vi "lib Compare Files in Folder.vi"() -> ()   [LabVIEW 2011]
panel:
  out "Array":T1(array[cluster])
  out "Horizontal Graduated Bar":u8(slide) scale=0.0..100.0
  out "All Files in Dir":path[](array[path])
  in  "Folder Path 2":path
  in  "Folder Path":path
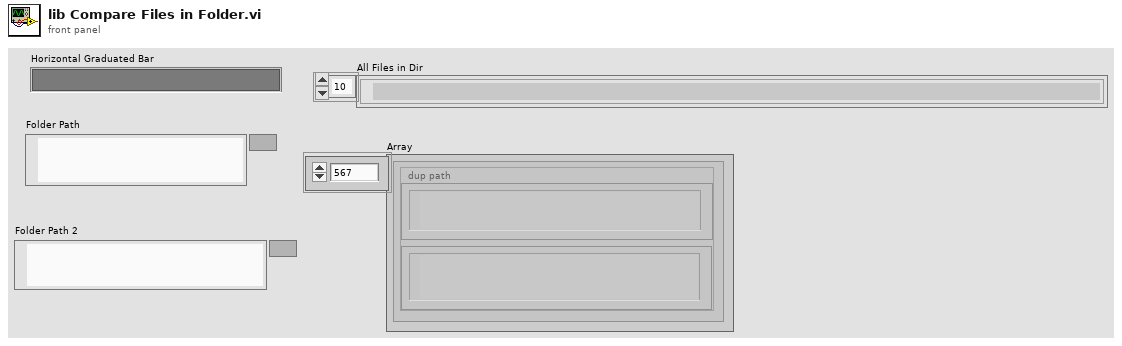
[diagram p1: front panel]
types:
  T1 = cluster{"dup path":path, "File Path Control":path}[]
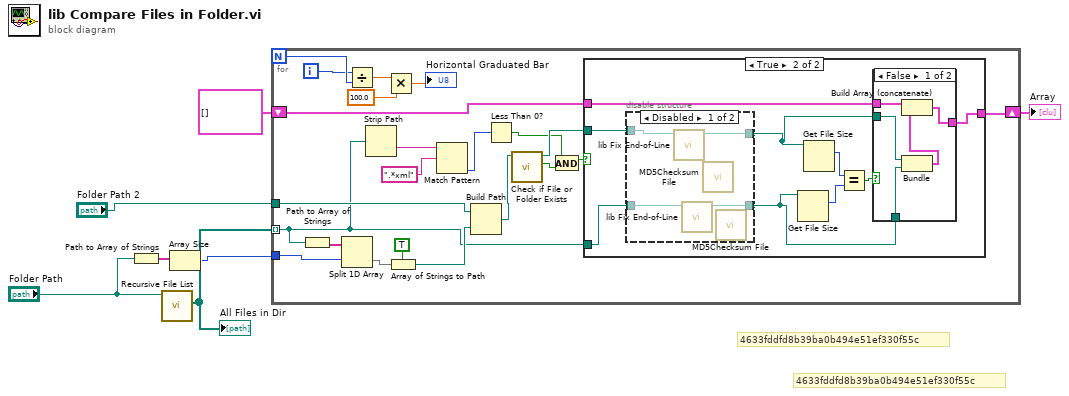
[diagram p0: block diagram]
diagram:
  # "4633fddfd8b39ba0b494e51ef330f55c"
  # "4633fddfd8b39ba0b494e51ef330f55c"
  n1 = Path to Array of Strings(0:"Folder Path") -> (2:w4:string[])  [unwired: 1 out]
  n2 = call <vilib>:"Recursive File List.vi"("Folder Path"="Folder Path") -> ("All Files in Dir"=w6:path[])  [unwired: 6 in, 4 out]
  "All Files in Dir" <- w6
  n3 = Array Size(array=w4) -> (size(s)=w3:i32)
  n4 = for {
    N -> [w18]
    tunnel: "Folder Path 2" -> [w25]
    tunnel: w6 -> [w13] mode=indexing
    tunnel: w3 -> [w28]
    shift-right: [w20] -> w1
    shift-left: cluster{"dup path":path, path}[] [] -> [w19]
    i -> [w17]
    n5 = Path to Array of Strings(0:w13) -> (2:w29:string[])  [unwired: 1 out]
    n6 = Split 1D Array(array=w29, index=w28) -> (second subarray=w27:string[])  [unwired: 1 out]
    n7 = Divide(x=w17, y=w18) -> (x/y=w16:dbl)
    n8 = Strip Path(path=w13) -> (name=w12:string)  [unwired: 1 out]
    n9 = Multiply(x=w16, y=100.0) -> (x*y=→"Horizontal Graduated Bar":dbl)
    n10 = Array of Strings to Path(0:w27, 1:TRUE ("relative")) -> (2:w24:path)
    n11 = Match Pattern(string=w12, regular expression=".*xml") -> (offset past match=w10:i32)  [unwired: 1 in, 3 out]
    n12 = Build Path(base path=w25, name or relative path=w24) -> (appended path=w23:path)
    n13 = Less Than 0?(x=w10) -> (x < 0?=w8:bool)
    n14 = call <vilib>:"Check if File or Folder Exists.vi"("path"=w23) -> ("file or folder exists?"=w22:bool, "dup path"=w21:path)  [unwired: 8 in, 1 out]
    n15 = And(x=w8, y=w22) -> (x .and. y?=w9:bool)
    n16 = case shown="True" w9 {
      tunnel: w21 -> [_ w35]
      tunnel: w13 -> [_ w36]
      tunnel: [w30 w38] -> w20
      tunnel: w19 -> [w30 w37]
      frame False {
      }
      frame True {
        n17 = disable-structure shown="Disabled" {
          disable-tunnel: w36 -> [w43 w44]
          disable-tunnel: [w42 w44] -> w33
          disable-tunnel: w35 -> [w41 w45]
          disable-tunnel: [w40 w45] -> w34
          frame Disabled {
            n18 = call "lib Fix End-of-Line.vi"("File"=w41) -> ("File dup"=w40:path)  [unwired: 9 in, 1 out]
            n19 = call "lib Fix End-of-Line.vi"("File"=w43) -> ("File dup"=w42:path)  [unwired: 9 in, 1 out]
            n20 = call <vilib>:"MD5Checksum File.vi"() -> ()  [unwired: 10 in, 2 out]
            n21 = call <vilib>:"MD5Checksum File.vi"() -> ()  [unwired: 10 in, 2 out]
          }
          frame Enabled {
          }
        }
        n22 = Get File Size(file=w33) -> (size (in bytes)=w32:i64)  [unwired: 1 in, 2 out]
        n23 = Get File Size(file=w34) -> (size (in bytes)=w31:i64)  [unwired: 1 in, 2 out]
        n24 = Equal?(x=w31, y=w32) -> (x = y?=w39:bool)
        n25 = case shown="False" w39 {
          tunnel: w34 -> [w48 _]
          tunnel: [w50 w51] -> w38
          tunnel: w37 -> [w49 w51]
          tunnel: w33 -> [w47 _]
          frame False {
            n26 = Bundle("dup path"=w48, w47) -> (w46:cluster{"dup path":path, path})  [unwired: 1 in]
            n27 = Build Array (concatenate)(w49, w46) -> (w50:cluster{"dup path":path, path}[])
          }
          frame True {
          }
        }
      }
    }
  }
  "Array" <- w1
